vi "DuplicateNode.vi"(7 "same parent?":bool, 8 "error in":errorcluster, 10 "new parent":T1, 11 "node ref in":T1) -> (0 "error out":errorcluster, 3 "new node ref":T1)   [LabVIEW 2013, in "NISE_CEF_TreeControl.lvlib"]
doc: "This VI duplicates a creates duplicate of a node.\nIf same parent is set to true the new node will use current parent, if set to false it will be added to the parent specified in the new parent terminal"
uses:
  NISE_CEF_TreeControl.lvlib
  Node/NodeRef.ctl
  Node/NISE_CEF_Node.lvclass
  Node/NISE_CEF_Node.lvclass/NISE_CEF_Node.ctl
  Node/ReadParent.vi
  Node/ReadChildren.vi
  Node/WriteChildren.vi
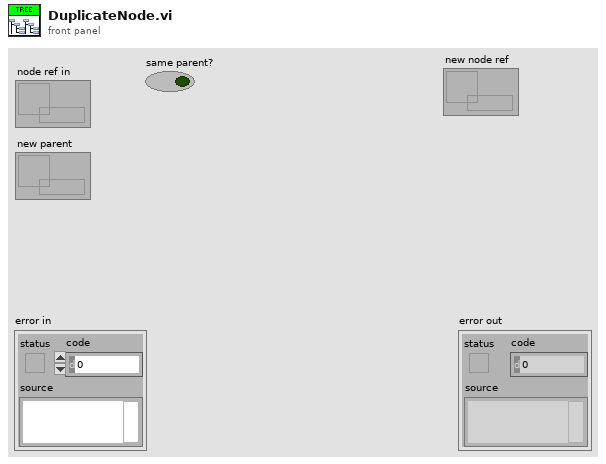
[diagram p1: front panel]
types:
  T1 = typedef "NISE_CEF_Node.lvclass/NodeRef.ctl" = refnum<data-value>
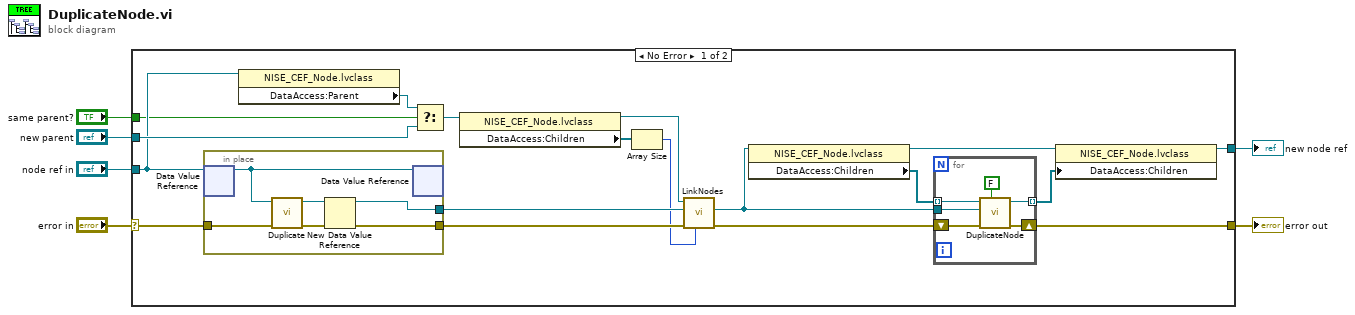
[diagram p0: block diagram]
diagram:
  n1 = case shown="No Error" "error in" {
    selector: "error in" -> [w13 w37]
    tunnel: [w22 w37] -> w5
    tunnel: "node ref in" -> [w20 _]
    tunnel: [w14 _] -> w3
    tunnel: "new parent" -> [w24 _]
    tunnel: "same parent?" -> [w7 _]
    frame No Error {
      n2 = in-place {
        in-place-border: [w36] -> w19
        in-place-border: w13 -> [w33]
        in-place-border: [w31] -> w12
        n3 = in-place-dvr #1(w20) -> (w35:refnum<class "NISE_CEF_Node.lvclass">)  [unwired: 1 out]
        n4 = call-dynamic "Duplicate.vi"("error in"=w33, "node in"=w35) -> ("error out"=w32:errorcluster, "node copy out"=w34:refnum<class "NISE_CEF_Node.lvclass">)  [unwired: 8 in]
        n5 = New Data Value Reference(data value=w34, error in=w32) -> (data value reference=w36:refnum<data-value>, error out=w31:errorcluster)
        n6 = in-place-dvr #1(w35) -> ()  [unwired: 2 out]
      }
      n7 = property class="NISE_CEF_Node.lvclass"(reference=w20) -> ("DataAccess:Parent"=w21:T1)  [unwired: 1 in, 2 out]
      n8 = Select(t=w21, s=w7, f=w24) -> (s? t:f=w11:T1)
      n9 = property class="NISE_CEF_Node.lvclass"(reference=w11) -> (reference out=w10:T1, "DataAccess:Children"=w9:T1[])  [unwired: 1 in, 1 out]
      n10 = Array Size(array=w9) -> (size(s)=w8:i32)
      n11 = call "LinkNodes.vi"("index"=w8, "error in"=w12, "child in"=w19, "parent in"=w10) -> ("error out"=w23:errorcluster, "child out"=w15:T1)  [unwired: 5 in, 1 out]
      n12 = property class="NISE_CEF_Node.lvclass"(reference=w15) -> (reference out=w18:T1, "DataAccess:Children"=w17:T1[])  [unwired: 1 in, 1 out]
      n13 = for {
        tunnel: w17 -> [w30] mode=indexing
        tunnel: [w29] -> w16 mode=indexing
        tunnel: w15 -> [w28]
        shift-right: [w26] -> w22
        shift-left: w23 -> [w27]
        n14 = call "DuplicateNode.vi"("same parent?"=FALSE ("s"), "error in"=w27, "new parent"=w28, "node ref in"=w30) -> ("error out"=w26:errorcluster, "new node ref"=w29:T1)  [unwired: 6 in]
      }
      n15 = property class="NISE_CEF_Node.lvclass"(reference=w18, "DataAccess:Children"=w16) -> (reference out=w14:T1)  [unwired: 1 in, 1 out]
    }
    frame Error {
    }
  }
  "error out" <- w5
  "new node ref" <- w3
